vi "DevicesSearch.vi"() -> (0 "devices":cluster{"DeviceName":string, "LocID":u32}[](array[cluster]))   [LabVIEW 2010]
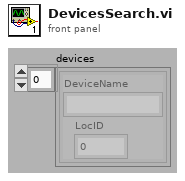
[diagram p1: front panel]
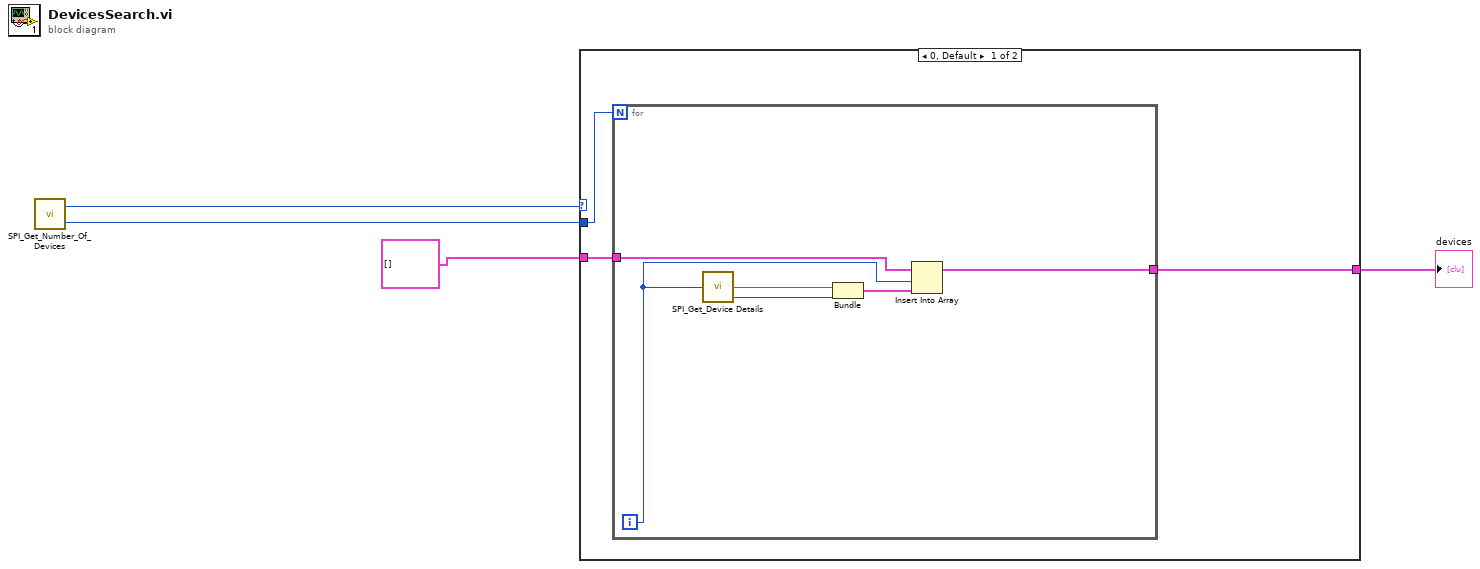
[diagram p0: block diagram]
diagram:
  n1 = call "SPI_Get_Number_Of_Devices.vi"() -> ("NumDevices"=w3:u32, "FTC_Status"=w4:u32)
  n2 = case shown="0, Default" w4 {
    tunnel: w3 -> [w7 _]
    tunnel: cluster{"DeviceName":string, "LocID":u32}[] [] ("array") -> [w6 _]
    tunnel: [w5 _] -> w1
    frame 0, Default {
      n3 = for {
        N: w7 -> [_]
        tunnel: w6 -> [w9]
        tunnel: [w8] -> w5
        i -> [w10]
        n4 = call "SPI_Get_Device Details.vi"("DeviceIndex"=w10) -> ("DeviceName"=w13:string, "LocID"=w12:u32)  [unwired: 1 out]
        n5 = Bundle("DeviceName"=w13, "LocID"=w12) -> (w11:cluster{"DeviceName":string, "LocID":u32})  [unwired: 1 in]
        n6 = Insert Into Array(array=w9, index=w10, new element=w11) -> (w8:cluster{"DeviceName":string, "LocID":u32}[])
      }
    }
    frame 1 {
    }
  }
  "devices" <- w1
